vi "RP-GET IP ADDRESS.vi"(1 "MAC address":string="00-26-32-F0-8D-DC") -> (0 "IP address":string)   [LabVIEW 2021]
uses:
  <vilib>/regexp/Match Regular Expression.xnode
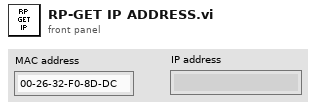
[diagram p1: front panel]
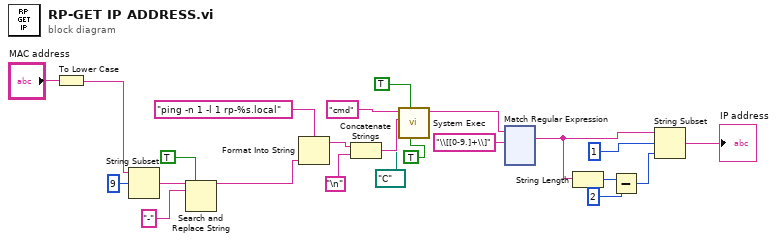
[diagram p0: block diagram]
diagram:
  n1 = To Lower Case(string="MAC address") -> (all lower case string=w22:string)
  n2 = String Subset(string=w22, offset (0)=9) -> (substring=w13:string)  [unwired: 1 in]
  n3 = Search and Replace String(replace all?=TRUE ("replace all? (F)"), input string=w13, search string="-") -> (result string=w11:string)  [unwired: 5 in, 3 out]
  n4 = Format Into String(format string="ping -n 1 -l 1 rp-%s.local", w11) -> (resulting string=w18:string)  [unwired: 2 in, 1 out]
  n5 = Concatenate Strings(w18, "\n") -> (w17:string)
  n6 = call <vilib>:"System Exec.vi"("run minimized? (F)"=TRUE, "wait until completion? (T)"=TRUE, "working directory"=path "C:/", "standard input"=w17, "command line"="cmd") -> ("standard output"=w6:string)  [unwired: 3 in, 3 out]
  n7 = xnode "Match Regular Expression"("input string"=w6, "regular expression"="\\[[0-9.]+\\]") -> ("whole match"=w4:string)  [unwired: 4 in, 4 out]
  n8 = String Length(string=w4) -> (length=w3:i32)
  n9 = Subtract(x=w3, y=2) -> (x-y=w1:i32)
  n10 = String Subset(string=w4, offset (0)=1, length (rest)=w1) -> (substring=→"IP address":string)
